vi "WireReadBlockDiagram.vi"(8 "error in":errorcluster, 10 "Terminal References":T4, 11 "State":T1) -> (0 "error out":errorcluster, 3 "State out":T1)   [LabVIEW 2013, in "data interface script.lvlib"]
uses:
  data interface script.lvlib
  Controls/TerminalReferences.ctl
  Controls/StateCluster.ctl
  Controls/initialized references.ctl
  Controls/interface VI type.ctl
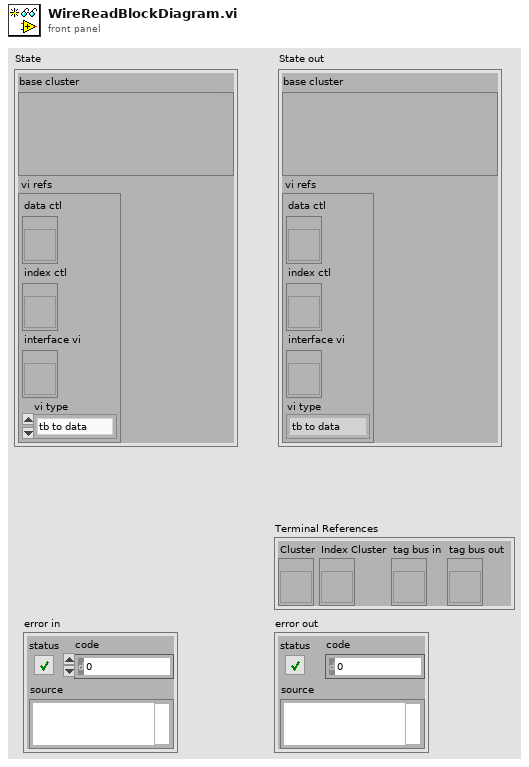
[diagram p1: front panel]
types:
  T1 = typedef "data interface script.lvlib/StateCluster.ctl" = cluster{"base cluster":variant, "vi refs":T2}
  T2 = typedef "data interface script.lvlib/initialized references.ctl" = cluster{"data ctl":refnum<vi>, "index ctl":refnum<vi>, "interface vi":refnum<vi>, "vi type":T3}
  T3 = typedef "data interface script.lvlib/interface VI type.ctl" = enum16{"tb to data", "data to tb"}
  T4 = typedef "data interface script.lvlib/TerminalReferences.ctl" = cluster{"Cluster":refnum<vi>, "Index Cluster":refnum<vi>, "tag bus in":refnum<vi>, "tag bus out":refnum<vi>}
  T5 = typedef "tag bus.lvlib/tag descriptor.lvclass/Data Type.ctl" = enum16{"Double", "Single", "I64", "I32", "I16", "I8", "U64", "U32", "U16", "U8", "Boolean", "String", "Array of Double", "Array of Single", "Array of I64", "Array of I32", "Array of I16", "Array of I8", "Array of U64", "Array of U32", "Array of U16", "Array of U8", "Array of Boolean", "Array of String"}
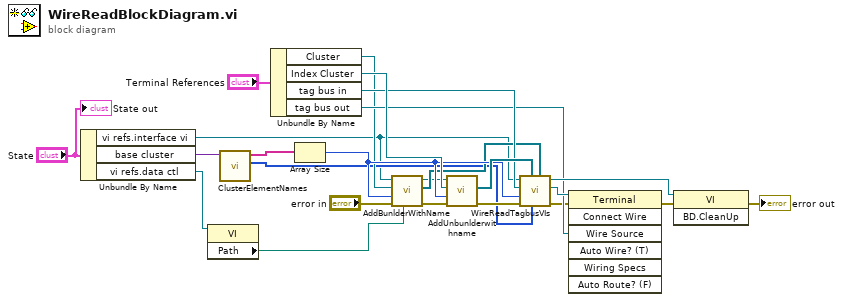
[diagram p0: block diagram]
diagram:
  n1 = Unbundle By Name("State") -> ("vi refs.interface vi"=w4:refnum<vi>, "base cluster"=w20:variant, "vi refs.data ctl"=w6:refnum<vi>)
  n2 = property class="VI"(reference=w6) -> ("Path"=w2:path)  [unwired: 1 in, 2 out]
  n3 = call "ClusterElementNames.vi"("input cluster"=w20) -> ("DataTypes"=w5:T5[], "Elements Names"=w19:string[])  [unwired: 8 in, 1 out]
  n4 = Unbundle By Name("Terminal References") -> ("Cluster"=w8:refnum<vi>, "Index Cluster"=w22:refnum<vi>, "tag bus in"=w17:refnum<vi>, "tag bus out"=w13:refnum<vi>)
  n5 = Array Size(array=w19) -> (size(s)=w11:i32)
  n6 = call "AddBunlderWithName.vi"("Cluster Path"=w2, "error in"="error in", "elements in cluster"=w11, "cluster terminal"=w8, "VI in"=w4) -> ("error out"=w7:errorcluster, "terminals"=w10:refnum<vi>[], "VI out"=w9:refnum<vi>)  [unwired: 4 in]
  n7 = call "AddUnbunlderwithname.vi"("error in"=w7, "elements in cluster"=w11, "cluster terminal"=w22, "VI in"=w9) -> ("error out"=w12:errorcluster, "terminals"=w21:refnum<vi>[])  [unwired: 5 in, 1 out]
  n8 = call "WireReadTagbusVIs.vi"("terminals data"=w10, "DataTypes"=w5, "terminals indexes"=w21, "error in"=w12, "elements in cluster"=w11, "tag bus in in"=w17, "VI in"=w4) -> ("error out"=w1:errorcluster, "tag bus out"=w14:refnum<vi>, "VI out"=w16:refnum<vi>)  [unwired: 2 in]
  n9 = invoke on="Invoke Node" class="Terminal" method="Connect Wire"(reference=w14, error in=w1, "Wire Source"=w13) -> (error out=w15:errorcluster)  [unwired: 4 in, 6 out]
  n10 = invoke class="VI" method="BD.CleanUp"(reference=w16, error in=w15) -> (error out=→"error out":errorcluster)  [unwired: 1 in, 2 out]
  "State out" <- "State"
